vi "Determine Test Graphs.vi"(6 "force":dbl[](array[numeric]), 7 "setpoint":dbl[](array[numeric]), 9 "force time":dbl[](array[numeric]), 10 "diameter":dbl[](array[numeric]), 11 "diameter time":dbl[](array[numeric])) -> (2 "force graph":T1(array[cluster]), 3 "diameter graph":T1(array[cluster]))   [LabVIEW 2020]
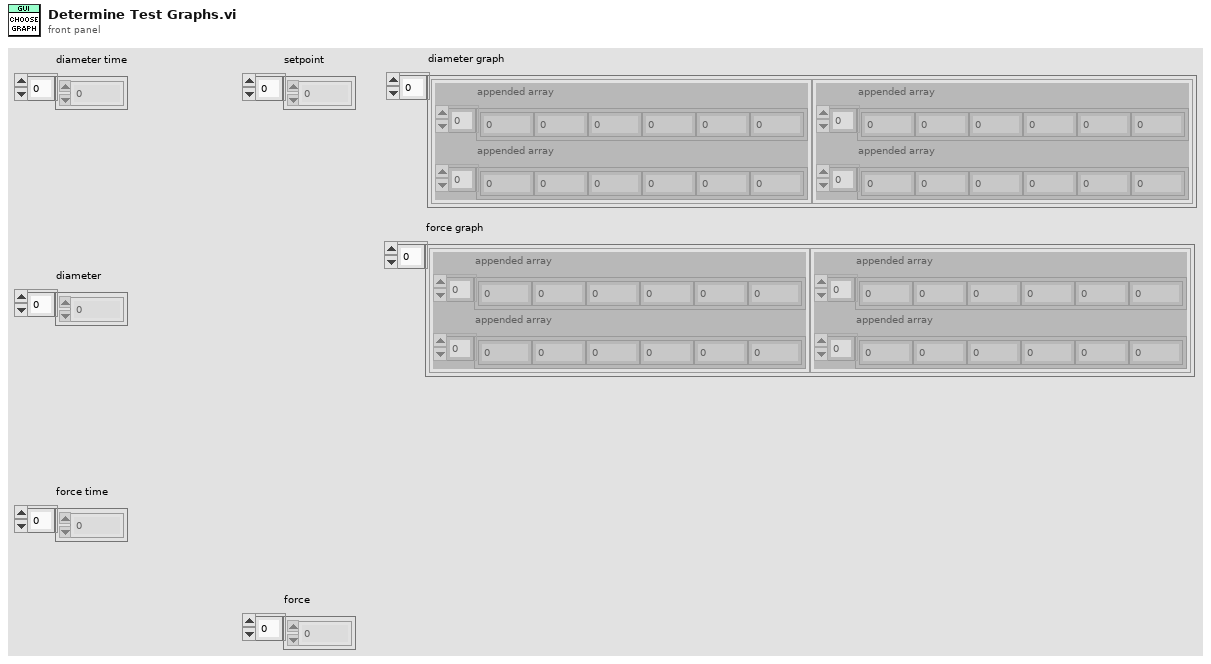
[diagram p1: front panel]
types:
  T1 = cluster{"appended array":dbl[], "appended array":dbl[]}[]
  T2 = cluster{"diameter time":dbl[], "diameter":dbl[]}[]
  T3 = cluster{"diameter time":dbl[], "setpoint":dbl[]}[]
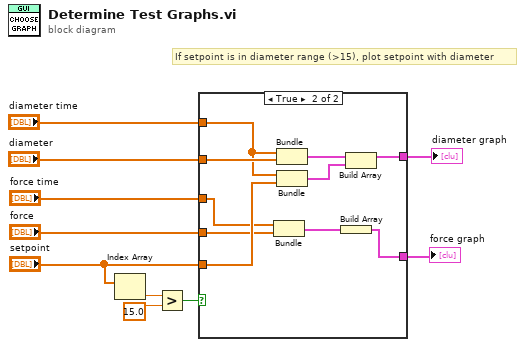
[diagram p0: block diagram]
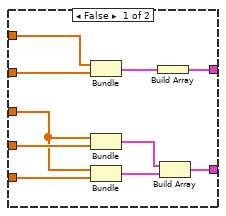
[diagram p2: hidden frame]
diagram:
  # "If setpoint is in diameter range (>15), plot setpoint with diameter"
  n1 = Index Array(array="setpoint") -> (element=w3:dbl)  [unwired: 1 in]
  n2 = Greater?(x=w3, y=15.0) -> (0:w1:bool)
  n3 = case shown="True" w1 {
    tunnel: [w20 w25] -> w10
    tunnel: "diameter" -> [w18 w28]
    tunnel: "diameter time" -> [w17 w27]
    tunnel: "force" -> [w16 w22]
    tunnel: "force time" -> [w15 w23]
    tunnel: [w12 w21] -> w5
    tunnel: "setpoint" -> [w11 w26]
    frame False {
      n4 = Bundle("diameter time"=w17, "diameter"=w18) -> (w19:cluster{"diameter time":dbl[], "diameter":dbl[]})  [unwired: 1 in]
      n5 = Bundle("force time"=w15, "force"=w16) -> (w13:cluster{"force time":dbl[], "force":dbl[]})  [unwired: 1 in]
      n6 = Bundle("force time"=w15, "setpoint"=w11) -> (w14:cluster{"force time":dbl[], "setpoint":dbl[]})  [unwired: 1 in]
      n7 = Build Array(w19) -> (w20:T2)
      n8 = Build Array(w13, w14) -> (w12:cluster{"force time":dbl[], "setpoint":dbl[]}[])
    }
    frame True {
      n9 = Bundle("force time"=w23, "force"=w22) -> (w24:cluster{"force time":dbl[], "force":dbl[]})  [unwired: 1 in]
      n10 = Bundle("diameter time"=w27, "diameter"=w28) -> (w29:cluster{"diameter time":dbl[], "diameter":dbl[]})  [unwired: 1 in]
      n11 = Bundle("diameter time"=w27, "setpoint"=w26) -> (w30:cluster{"diameter time":dbl[], "setpoint":dbl[]})  [unwired: 1 in]
      n12 = Build Array(w24) -> (w21:cluster{"force time":dbl[], "force":dbl[]}[])
      n13 = Build Array(w29, w30) -> (w25:T3)
    }
  }
  "diameter graph" <- w10
  "force graph" <- w5
